vi "Servo Pulse Gen..vi"() -> ()   [LabVIEW 2015]
uses:
  Slide Servo.ctl
  Galobal variable_TI.vi
  Project Setup/Globle Variable/GR_Servo.vi
panel:
  out "Enum":T1
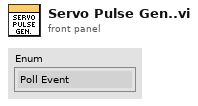
[diagram p1: front panel]
types:
  T1 = typedef "Slide Servo.ctl" = enum16{"Poll Event", "Servo CMD", "Slide Servo Home ", "Exit"}
  T2 = cluster{"Emergency":bool, "Air Pressure":bool, "Saftey Sensor":bool, "Slide Servo  fault":bool, "Reset":bool, "Pressing Cyl Up RS_AI19":bool}
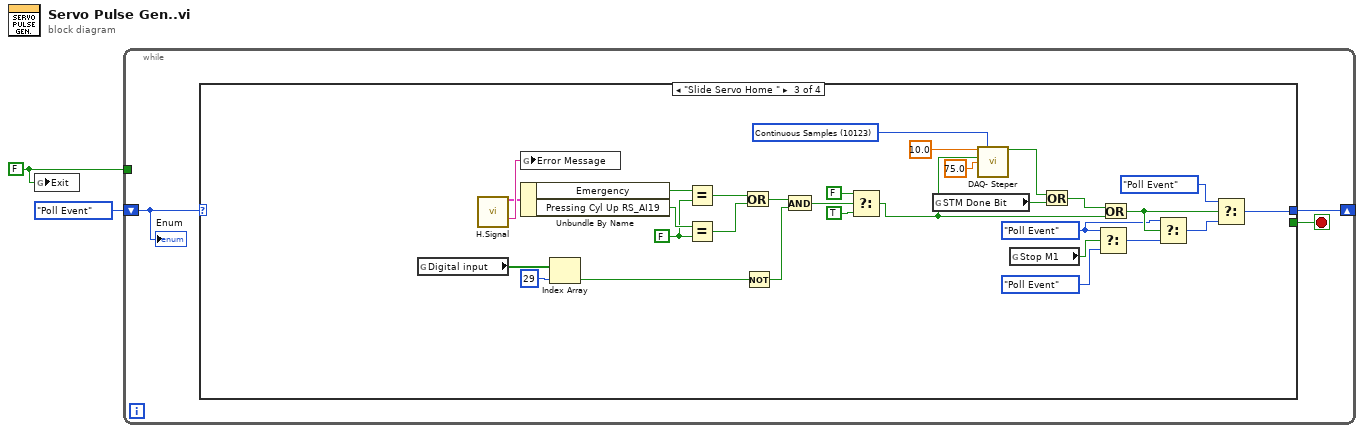
[diagram p0: block diagram]
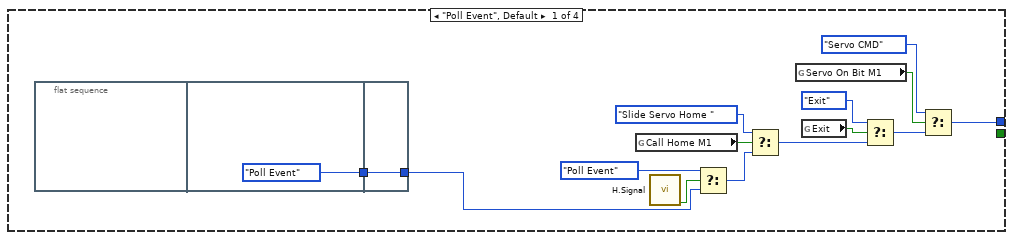
[diagram p2: hidden frame]
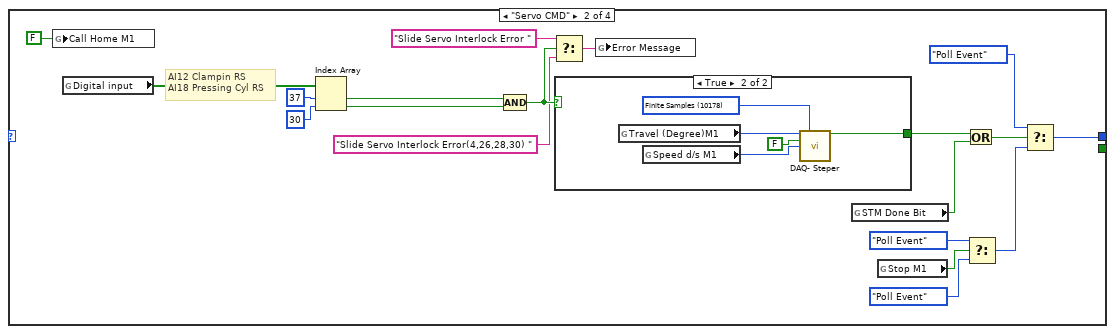
[diagram p3: hidden frame]
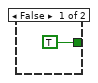
[diagram p4: hidden frame]
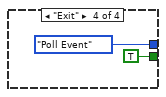
[diagram p5: hidden frame]
diagram:
  w1 = FALSE ("Exit")
  n1 = global write "Galobal variable_TI.vi" "Exit"(w1) -> ()
  n2 = while {
    shift-right: [w4] -> _
    shift-left: Slide_Servo."Poll Event" ("Enum") -> [w5]
    tunnel: w1 -> [_]
    stop <- w3 stop-if-true
    n3 = case shown="\"Slide Servo Home \"" w5 {
      tunnel: [w14 w36 w66 Slide_Servo."Poll Event" ("Enum")] -> w4
      tunnel: [_ _ _ TRUE] -> w3
      frame "Poll Event", Default {
        n4 = flat-sequence {
          tunnel: [Slide_Servo."Poll Event" ("Enum")] -> w6
          tunnel: [w21] -> w7
          tunnel: w6 -> [w21]
          frame #0 {
          }
          frame #1 {
          }
          frame #2 {
          }
        }
        n5 = global read "Galobal variable_TI.vi" "Call Home M1"() -> (w12:bool)
        n6 = call "H.Signal.vi"() -> ("Bool_H Sig"=w8:bool)  [unwired: 12 in, 3 out]
        n7 = Select(t=Slide_Servo."Poll Event" ("Enum"), s=w8, f=w7) -> (s? t:f=w9:T1)
        n8 = Select(t=Slide_Servo."Slide Servo Home " ("Enum"), s=w12, f=w9) -> (s? t:f=w11:T1)
        n9 = global read "GR_Servo.vi" "Servo On Bit M1"() -> (w17:bool)
        n10 = global read "Galobal variable_TI.vi" "Exit"() -> (w18:bool)
        n11 = Select(t=Slide_Servo."Exit" ("Enum"), s=w18, f=w11) -> (s? t:f=w19:T1)
        n12 = Select(t=Slide_Servo."Servo CMD" ("Enum"), s=w17, f=w19) -> (s? t:f=w14:T1)
      }
      frame "Servo CMD" {
        # "AI12 Clampin RS\nAI18 Pressing Cyl RS"
        n13 = global write "Galobal variable_TI.vi" "Call Home M1"(FALSE ("Call Home M1")) -> ()
        n14 = global read "Galobal variable_TI.vi" "Digital input"() -> (w30:bool[])
        n15 = Index Array(array=w30, index #1=37 ("index"), index #2=30 ("index")) -> (element #1=w26:bool, element #2=w27:bool)
        n16 = Compound Arithmetic op=AND(w26, w27) -> (w25:bool)
        n17 = Select(t="Slide Servo Interlock Error ", s=w25, f="Slide Servo Interlock Error(4,26,28,30) ") -> (s? t:f=w22:string)
        n18 = case shown="True" w25 {
          tunnel: [TRUE ("Task Done Bit") w44] -> w40
          frame False {
          }
          frame True {
            w42 = 10178 items=["Finite Samples"=10178, "Continuous Samples"=10123, "Hardware Timed Single Point"=12522] ("Mode")
            n19 = global read "GR_Servo.vi" "Travel (Degree)M1"() -> (w45:i32)
            n20 = global read "GR_Servo.vi" "Speed d/s M1"() -> (w46:i32)
            n21 = call "DAQ- Steper.vi"("Travel (Degree)"=w45, "Mode"=w42, "Home Condition"=FALSE, "Speed d/s"=w46) -> ("Task Done Bit"=w44:bool)  [unwired: 10 in, 1 out]
          }
        }
        n22 = global write "GR_Servo.vi" "Error Message"(w22) -> ()
        n23 = global read "Galobal variable_TI.vi" "STM Done Bit"() -> (w39:bool)
        n24 = global read "Galobal variable_TI.vi" "Stop M1"() -> (w35:bool)
        n25 = Or(x=w40, y=w39) -> (x .or. y?=w38:bool)
        n26 = Select(t=Slide_Servo."Poll Event" ("Enum"), s=w35, f=Slide_Servo."Poll Event" ("Enum")) -> (s? t:f=w32:T1)
        n27 = Select(t=Slide_Servo."Poll Event" ("Enum"), s=w38, f=w32) -> (s? t:f=w36:T1)
      }
      frame "Slide Servo Home " {
        w55 = FALSE ("y")
        w65 = 10123 items=["Finite Samples"=10178, "Continuous Samples"=10123, "Hardware Timed Single Point"=12522] ("Mode")
        w68 = Slide_Servo."Poll Event" ("Enum")
        n28 = global read "Galobal variable_TI.vi" "Digital input"() -> (w52:bool[])
        n29 = call "H.Signal.vi"() -> ("output cluster"=w61:T2, "Error Message"=w62:string)  [unwired: 12 in, 2 out]
        n30 = global write "GR_Servo.vi" "Error Message"(w62) -> ()
        n31 = Unbundle By Name(w61) -> ("Emergency"=w60:bool, "Pressing Cyl Up RS_AI19"=w56:bool)
        n32 = Index Array(array=w52, index=29) -> (element=w49:bool)
        n33 = Equal?(x=w60, y=w55) -> (x = y?=w53:bool)
        n34 = Equal?(x=w56, y=w55) -> (x = y?=w54:bool)
        n35 = Or(x=w53, y=w54) -> (x .or. y?=w50:bool)
        n36 = Not(x=w49) -> (.not. x?=w48:bool)
        n37 = And(x=w50, y=w48) -> (x .and. y?=w47:bool)
        n38 = Select(t=FALSE ("y"), s=w47, f=TRUE) -> (s? t:f=w58:bool)
        n39 = global read "Galobal variable_TI.vi" "STM Done Bit"() -> (w75:bool)
        n40 = call "DAQ- Steper.vi"("Travel (Degree)"=10.0, "Mode"=w65, "Home Condition"=w58, "Speed d/s"=75.0) -> ("Task Done Bit"=w76:bool)  [unwired: 10 in, 1 out]
        n41 = global read "Galobal variable_TI.vi" "Stop M1"() -> (w72:bool)
        n42 = Or(x=w76, y=w75) -> (x .or. y?=w73:bool)
        n43 = Select(t=w68, s=w72, f=Slide_Servo."Poll Event" ("Enum")) -> (s? t:f=w69:T1)
        n44 = Or(x=w73, y=w58) -> (x .or. y?=w70:bool)
        n45 = Select(t=w68, s=w70, f=w69) -> (s? t:f=w67:T1)
        n46 = Select(t=Slide_Servo."Poll Event" ("Enum"), s=w70, f=w67) -> (s? t:f=w66:T1)
      }
      frame "Exit" {
      }
    }
    "Enum" <- w5
  }
